vi "Main Hello World.vi"   [LabVIEW 2021]
uses:
  Hello World Queue/Hello World Queue/Hello World Queue.lvclass
  C:/git/jettl/src/jettl/Queue/Queue.lvclass
  jettl/jettl.lvlib
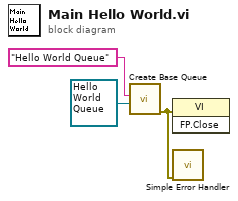
[diagram p0: block diagram]
diagram:
  n1 = call "Create Base Queue.vi"("Queue"=refnum<class "Hello World Queue.lvclass"> refnum ("Hello World Queue.lvlib:Hello World Queue.lvclass"), "Self Queue Alias"="Hello World Queue" ("Alias")) -> ("error out"=w1:errorcluster)  [unwired: 9 in]
  n2 = invoke class="VI" method="FP.Close"(error in=w1) -> ()  [unwired: 2 in, 3 out]
  n3 = call <vilib>:"Simple Error Handler.vi"("error in (no error)"=w1) -> ()  [unwired: 4 in, 5 out]
